vi "Draw Shapes.vi"(4 "Path Points":cluster{"x":dbl, "y":dbl}[](array[cluster]), 5 "Sample Period (s)":dbl=0.02, 6 "Output Point":T3, 7 "Commands":cluster{"Time (s)":dbl, T1, "Enabled":bool}[](array[cluster]), 8 "Results":T4, 9 "new picture in":picture, 10 "Points":cluster{"x":dbl, "y":dbl, "th":dbl}[](array[cluster]), 11 "Picture in":refnum<vi>) -> (3 "new picture out":picture)   [LabVIEW 2019]
uses:
  Command Stuff/Single Cmd Info.ctl
  <vilib>/picture/picture.llb/imagedata.ctl
  Globals.vi
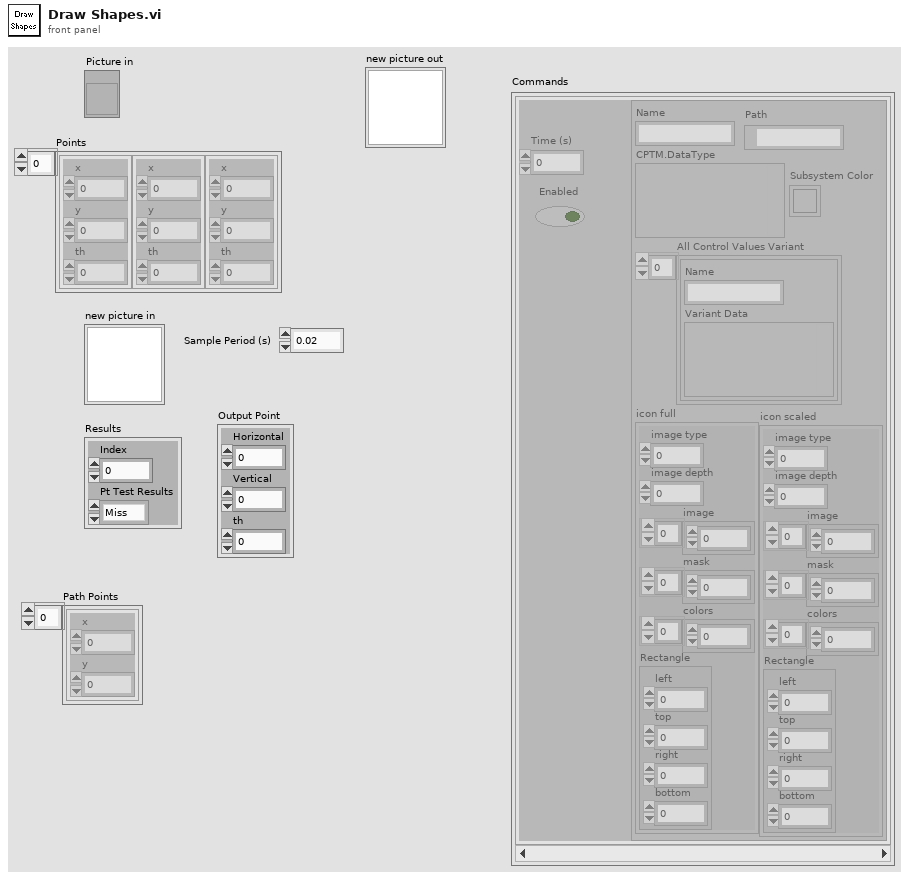
[diagram p1: front panel]
types:
  T1 = typedef "Single Cmd Info.ctl" = cluster{"Name":string, "CPTM.DataType":variant, "All Control Values Variant":cluster{"Name":string, "Variant Data":variant}[], "icon full":T2, "icon scaled":T2, "Path":path, "Subsystem Color":u32}
  T2 = typedef "imagedata.ctl" = cluster{"image type":i32, "image depth":i32, "image":u8[], "mask":u8[], "colors":u32[], "Rectangle":cluster{"left":i16, "top":i16, "right":i16, "bottom":i16}}
  T3 = cluster{"Horizontal":dbl, "Vertical":dbl, "th":dbl}
  T4 = cluster{"Index":i32, "Pt Test Results":enum16{"Miss", "Rect Hit", "Arrow Hit"}}
  T5 = typedef "LVPositionTypeDef.ctl" = cluster{"Left":i32, "Top":i32}
  T6 = typedef "LVBoundsTypeDef.ctl" = cluster{"Width":u32, "Height":u32}
  T7 = cluster{"left":i16, "top":i16, "right":i16, "bottom":i16}
  T8 = cluster{"Horizontal":dbl, "Vertical":dbl, "Horizontal":dbl, "Vertical":dbl}
  T9 = cluster{i32, "Pt Test Results":enum16{"Miss", "Rect Hit", "Arrow Hit"}}
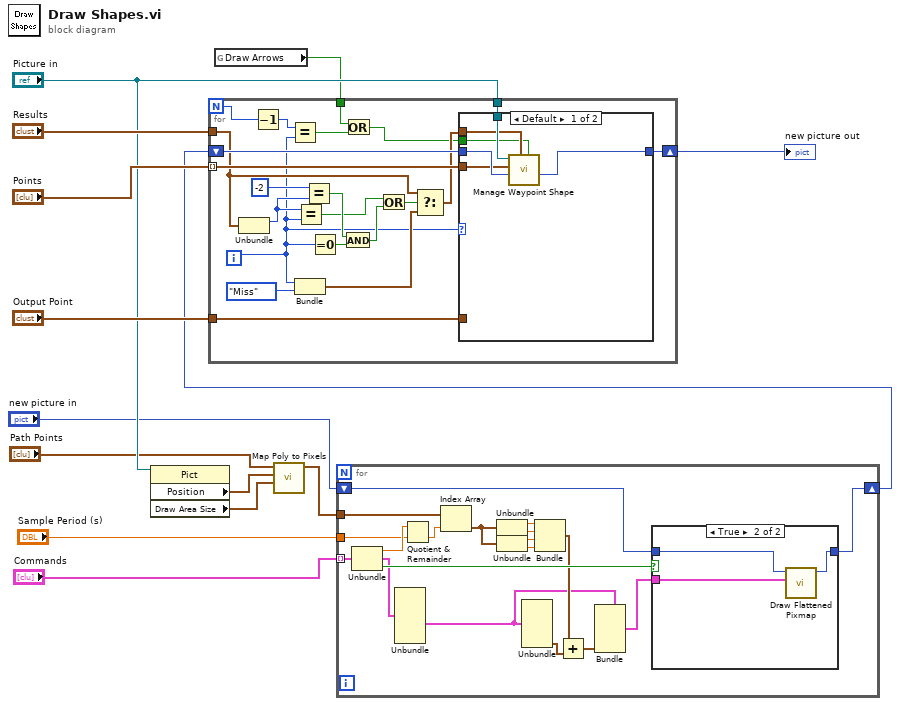
[diagram p0: block diagram]
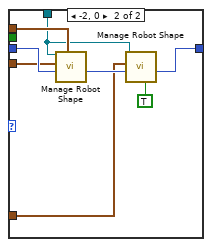
[diagram p3: hidden frame]
diagram:
  n1 = property on="Property Node" class="Pict"(reference="Picture in") -> ("Position"=w8:T5, "Draw Area Size"=w9:T6)  [unwired: 1 in, 2 out]
  n2 = global read "Globals.vi" "Draw Arrows"() -> (w1:bool)
  n3 = call "Map Poly to Pixels.vi"("Draw Area Size"=w9, "Position"=w8, "Coords"="Path Points") -> ("Coords"=w6:cluster{"Horizontal":dbl, "Vertical":dbl}[])  [unwired: 8 in]
  n4 = for {
    shift-right: [w26] -> w3
    shift-left: "new picture in" -> [w28]
    tunnel: "Commands" -> [w33] mode=indexing
    tunnel: w6 -> [w32]
    tunnel: "Sample Period (s)" -> [w30]
    n5 = Unbundle(w33) -> ("Time (s)"=w31:dbl, w24:T1, "Enabled"=w27:bool)
    n6 = Unbundle(w24) -> ("icon scaled"=w16:T2)  [unwired: 6 out]
    n7 = Quotient & Remainder(x=w31, y=w30) -> (floor(x/y)=w29:dbl)  [unwired: 1 out]
    n8 = Index Array(array=w32, index=w29) -> (element=w15:cluster{"Horizontal":dbl, "Vertical":dbl})
    n9 = Unbundle(w15) -> ("Horizontal"=w23:dbl, "Vertical"=w22:dbl)
    n10 = Unbundle(w15) -> ("Horizontal"=w21:dbl, "Vertical"=w20:dbl)
    n11 = Unbundle(w16) -> ("Rectangle"=w18:T7)  [unwired: 5 out]
    n12 = Bundle("Horizontal"=w23, "Vertical"=w22, "Horizontal"=w21, "Vertical"=w20) -> (w17:T8)  [unwired: 1 in]
    n13 = Add(x=w17, y=w18) -> (x+y=w25:cluster{dbl, dbl, dbl, dbl})
    n14 = Bundle(cluster=w16, "Rectangle"=w25) -> (w19:T2)  [unwired: 5 in]
    n15 = case shown="True" w27 {
      tunnel: [w34 w35] -> w26
      tunnel: w28 -> [w34 w36]
      tunnel: w19 -> [_ w37]
      frame False {
      }
      frame True {
        n16 = call <vilib>:"Draw Flattened Pixmap.vi"("image data"=w37, "picture"=w36) -> ("new picture"=w35:picture)  [unwired: 7 in]
      }
    }
  }
  n17 = for {
    N -> [w44]
    tunnel: "Points" -> [w59] mode=indexing
    shift-right: [w58] -> w2
    shift-left: w3 -> [w57]
    tunnel: "Picture in" -> [w56]
    tunnel: "Results" -> [w53]
    tunnel: "Output Point" -> [w41]
    tunnel: w1 -> [w38]
    i -> [w42]
    n18 = Unbundle(w53) -> ("Index"=w49:i32)  [unwired: 1 out]
    n19 = Decrement(x=w44) -> (x-1=w43:i32)
    n20 = Equal?(x=w43, y=w42) -> (x = y?=w40:bool)
    n21 = Bundle(w42, "Pt Test Results"=enum16{"Miss", "Rect Hit", "Arrow Hit"}."Miss") -> (w54:T9)  [unwired: 1 in]
    n22 = Equal?(x=w49, y=w42) -> (x = y?=w46:bool)
    n23 = Equal?(x=-2, y=w49) -> (x = y?=w48:bool)
    n24 = Equal To 0?(x=w42) -> (x = 0?=w51:bool)
    n25 = And(x=w48, y=w51) -> (x .and. y?=w47:bool)
    n26 = Or(x=w38, y=w40) -> (x .or. y?=w39:bool)
    n27 = Or(x=w46, y=w47) -> (x .or. y?=w45:bool)
    n28 = Select(t=w53, s=w45, f=w54) -> (s? t:f=w55:T4)
    n29 = case shown="Default" w42 {
      tunnel: w59 -> [w61 w72]
      tunnel: [w64 w69] -> w58
      tunnel: w57 -> [w65 w73]
      tunnel: w56 -> [w63 w67]
      tunnel: w55 -> [w62 w71]
      tunnel: w39 -> [w60 _]
      tunnel: w41 -> [_ w68]
      frame Default {
        n30 = call "Manage Waypoint Shape.vi"("Draw Arrow"=w60, "Drawing Options"=w62, "new picture in"=w65, "Waypoint Position (ft)"=w61, "Pict Ref"=w63) -> ("new picture out"=w64:picture)  [unwired: 5 in, 1 out]
      }
      frame -2, 0 {
        n31 = call "Manage Robot Shape.vi"("Drawing Options"=w71, "new picture in"=w73, "Robot Position (ft)"=w72, "Pict Ref"=w67) -> ("new picture out"=w70:picture)  [unwired: 5 in, 2 out]
        n32 = call "Manage Robot Shape.vi"("Lighter"=TRUE ("Outline"), "new picture in"=w70, "Robot Position (ft)"=w68, "Pict Ref"=w67) -> ("new picture out"=w69:picture)  [unwired: 5 in, 2 out]
      }
    }
  }
  "new picture out" <- w2
